vi "Parse Float Data Array.vi"(8 "error in (no error)":errorcluster, 10 "PLC Data in":T1, 11 "Data Read":u8[][](array[numeric])) -> (0 "error out":errorcluster, 2 "PLC Data out":T1, 5 "Motor2RatingRPM":u16, 7 "Motor1RatingRPM":u16)   [LabVIEW 2018]
uses:
  Ctls/DisplayIndicator.ctl
  Ctls/MotroConfigData.ctl
  Ctls/MotorConfig.ctl
  Ctls/MagType.ctl
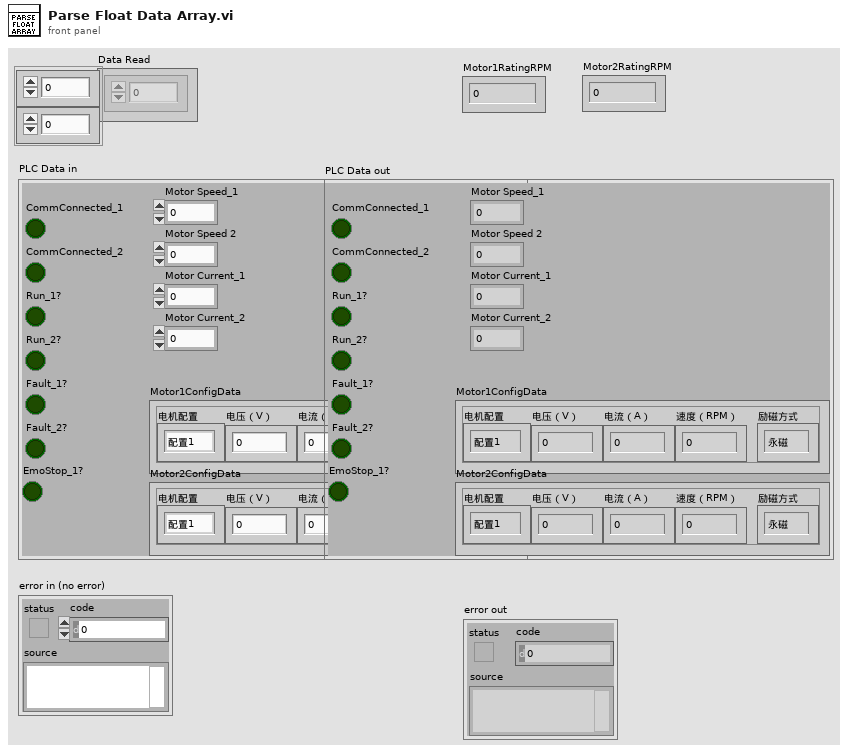
[diagram p1: front panel]
types:
  T1 = typedef "DisplayIndicator.ctl" = cluster{"CommConnected_1":bool, "Run_1?":bool, "Fault_1?":bool, "CommConnected_2":bool, "Run_2?":bool, "Fault_2?":bool, "Motor Speed 2":sgl, "Motor Speed_1":sgl, "Motor Current_1":sgl, "Motor Current_2":sgl, "Motor1ConfigData":T2, "Motor2ConfigData":T2, "EmoStop_1?":bool}
  T2 = typedef "MotroConfigData.ctl" = cluster{"电机配置":T3, "电压（V）":dbl, "电流（A）":dbl, "速度（RPM）":dbl, "励磁方式":T4}
  T3 = typedef "MotorConfig.ctl" = enum16{"配置1", "配置2", "配置3", "配置4"}
  T4 = typedef "MagType.ctl" = enum16{"永磁", "励磁"}
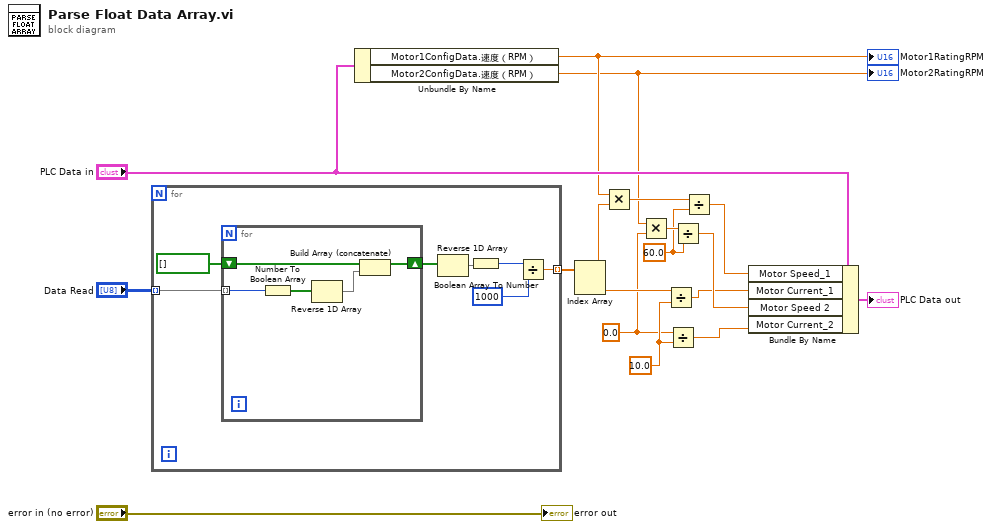
[diagram p0: block diagram]
diagram:
  w1 = 0.0 ("x")
  w3 = 10.0 ("y")
  w11 = 60.0 ("y")
  n1 = for {
    tunnel: "Data Read" -> [w25] mode=indexing
    tunnel: [w19] -> w15 mode=indexing
    n2 = for {
      tunnel: w25 -> [w30] mode=indexing
      shift-right: [w28] -> w23
      shift-left: bool[] [] ("Boolean array") -> [w29]
      n3 = Number To Boolean Array(number=w30) -> (Boolean array=w27:bool[])
      n4 = Reverse 1D Array(array=w27) -> (reversed array=w26:bool[])
      n5 = Build Array (concatenate)(w29, w26) -> (w28:bool[])
    }
    n6 = Reverse 1D Array(array=w23) -> (reversed array=w22:bool[])
    n7 = Boolean Array To Number(Boolean array=w22) -> (number=w21:u32)
    n8 = Divide(x=w21, y=u16 1000) -> (x/y=w19:dbl)
  }
  n9 = Unbundle By Name("PLC Data in") -> ("Motor1ConfigData.速度（RPM）"=w7:dbl, "Motor2ConfigData.速度（RPM）"=w6:dbl)
  "Motor1RatingRPM" <- w7
  "Motor2RatingRPM" <- w6
  n10 = Index Array(array=w15) -> (element #1=w14:dbl, element #2=w5:dbl)  [unwired: 2 in]
  n11 = Multiply(x=w7, y=w14) -> (x*y=w12:dbl)
  n12 = Multiply(x=w6, y=w1) -> (x*y=w13:dbl)
  n13 = Divide(x=w5, y=w3) -> (x/y=w4:dbl)
  n14 = Divide(x=w1, y=w3) -> (x/y=w2:dbl)
  n15 = Divide(x=w13, y=w11) -> (x/y=w10:dbl)
  n16 = Divide(x=w12, y=w11) -> (x/y=w9:dbl)
  n17 = Bundle By Name(cluster="PLC Data in", "Motor Speed_1"=w9, "Motor Current_1"=w4, "Motor Speed 2"=w10, "Motor Current_2"=w2) -> (→"PLC Data out":T1)
  "error out" <- "error in (no error)"
